vi "get distance order.vi"(5 "Overwrite Lib Path":path, 8 "error in (no error)":errorcluster) -> (0 "error out":errorcluster, 3 "Minkowski Distance Order":i32)   [LabVIEW 2020, in "KD Tree.lvlib"]
doc: "Gets the distance order in use throughout FLANN (only applicable if minkowski distance\n * is in use)."
uses:
  KD Tree.lvlib
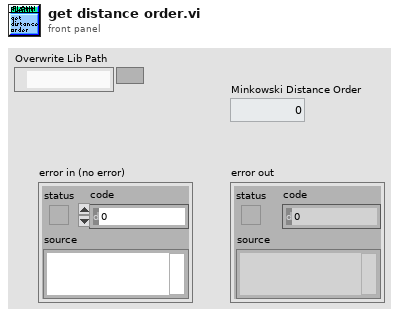
[diagram p1: front panel]
types:
  T1 = typedef "Semaphore RefNum" = refnum<k1>
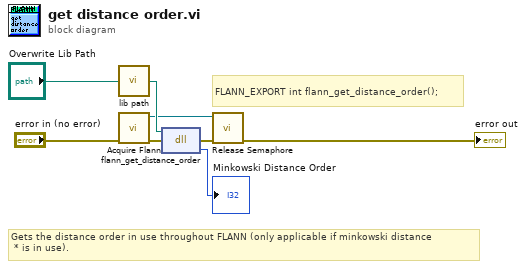
[diagram p0: block diagram]
diagram:
  # "Gets the distance order in use throughout FLANN (only applicable if minkowski distance\n * is in use)."
  # "FLANN_EXPORT int flann_get_distance_order();"
  n1 = call "lib path.vi"("Overwrite Lib Path"="Overwrite Lib Path") -> ("lib path"=w6:path)
  n2 = call "Acquire Flann.vi"("error in (no error)"="error in (no error)") -> ("error out"=w1:errorcluster, "semaphore"=w3:T1)  [unwired: 9 in]
  n3 = dll-call lib="E:/Labview/LV 2020/Libs/flann/flann.*" fn="flann_get_distance_order"(path in=w6, error in=w1) -> (error out=w7:errorcluster, "return type"=→"Minkowski Distance Order":i32)  [unwired: 1 in, 1 out]
  n4 = call <vilib>:"Release Semaphore.vi"("error in (no error)"=w7, "semaphore"=w3) -> ("error out"=→"error out":errorcluster)  [unwired: 4 in, 1 out]
